vi "Get Main Path.vi"(8 "Error In":errorcluster) -> (0 "Error Out":errorcluster, 2 "Main Name":string, 3 "Main Dir":path)   [LabVIEW 2011, in "LMH-Toolbox.lvlib"]
doc: "Get the directory containing the the main VI if running in the development environment or the exe if running in the run-time."
uses:
  LMH-Toolbox.lvlib
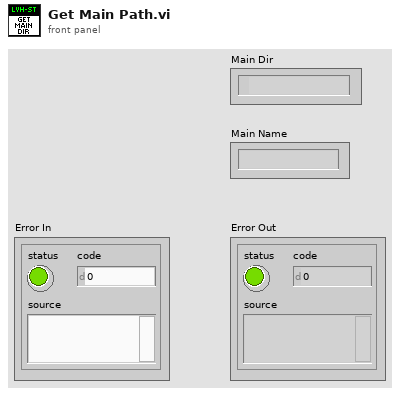
[diagram p1: front panel]
types:
  T1 = enum32{"invalid app kind", "Development System", "Run Time System", "Student Edition", "Embedded LabVIEW", "Evaluation", "Custom"}
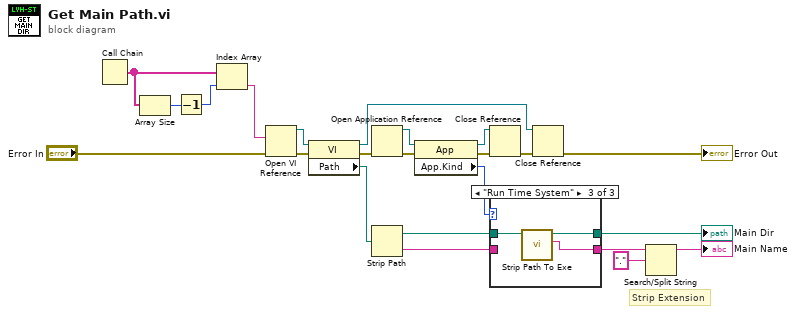
[diagram p0: block diagram]
diagram:
  # "Strip Extension"
  n1 = Call Chain() -> (call chain=w20:string[])
  n2 = Array Size(array=w20) -> (size(s)=w18:i32)
  n3 = Decrement(x=w18) -> (x-1=w19:i32)
  n4 = Index Array(array=w20, index=w19) -> (element=w23:string)
  n5 = Open VI Reference(vi path=w23, error in (no error)="Error In") -> (vi reference=w16:refnum<vi>, error out=w22:errorcluster)  [unwired: 4 in]
  n6 = property class="VI"(reference=w16, error in=w22) -> (reference out=w6:refnum<vi>, error out=w9:errorcluster, "Path"=w17:path)
  n7 = Open Application Reference(8:w9) -> (0:w8:errorcluster, 3:w15:refnum<vi>)  [unwired: 3 in]
  n8 = Strip Path(path=w17) -> (stripped path=w13:path, name=w4:string)
  n9 = property class="App"(reference=w15, error in=w8) -> (reference out=w7:refnum<vi>, error out=w12:errorcluster, "App.Kind"=w14:T1)
  n10 = Close Reference(reference=w7, error in (no error)=w12) -> (error out=w11:errorcluster)
  n11 = case shown="\"Run Time System\"" w14 {
    tunnel: [w25 w27 w29] -> w5
    tunnel: w13 -> [w25 w27 w30]
    tunnel: [w24 w26 w28] -> w3
    tunnel: w4 -> [w24 w26 _]
    frame "invalid app kind", Default {
    }
    frame "Development System" {
    }
    frame "Run Time System" {
      n12 = call "Strip Path To Exe.vi"("VI Path"=w30) -> ("exe Name"=w28:string, "exe Dir"=w29:path)  [unwired: 8 in, 1 out]
    }
  }
  "Main Dir" <- w5
  n13 = Close Reference(reference=w6, error in (no error)=w11) -> (error out=→"Error Out":errorcluster)
  n14 = Search/Split String(string=w3, search string/char (-)=".") -> (substring before match=→"Main Name":string)  [unwired: 1 in, 2 out]
